vi "GetWL.vi"(2 "error in (no error)":errorcluster, 3 "Integration Time":i32, 4 "Type":enum16{"Get Background", "Measure", "Raw"}(ring)=enum."Measure", 5 "USB4000 Params In":T1) -> (0 "error out":errorcluster, 1 "USB4000 Params Out":T1)   [LabVIEW 2012]
uses:
  Controls/USB4000_Data.ctl
panel:
  out "Array length":i32
  out "EL spectrum":dbl[](array[numeric])
  out "Wavelength":dbl[](array[numeric]) format="%.2f"
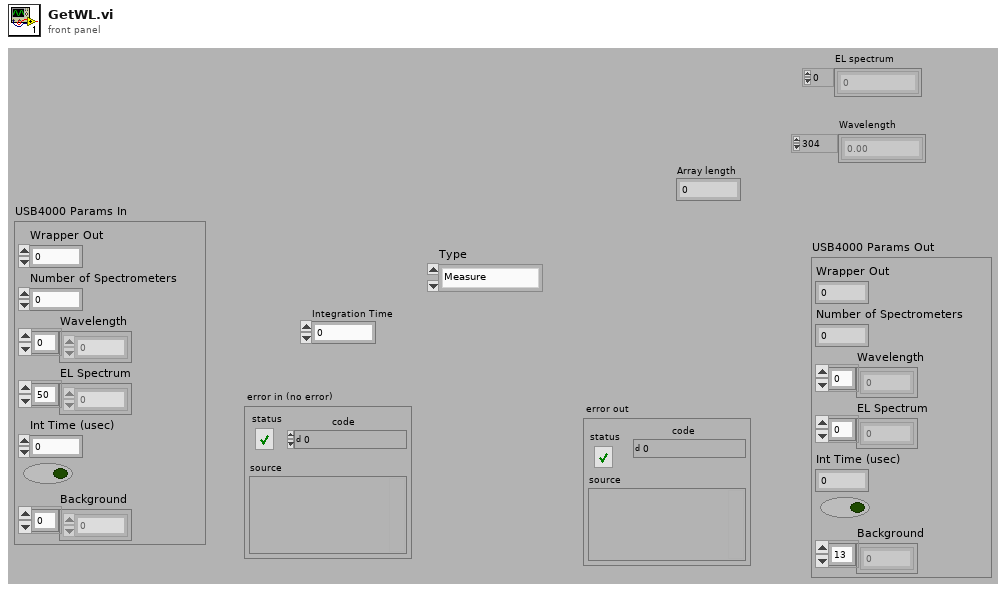
[diagram p1: front panel]
types:
  T1 = typedef "USB4000_Data.ctl" = cluster{"Wrapper Out":u32, "Number of Spectrometers":i32, "Wavelength":dbl[], "EL Spectrum":dbl[], "Int Time (usec)":i32, bool, "Background":dbl[]}
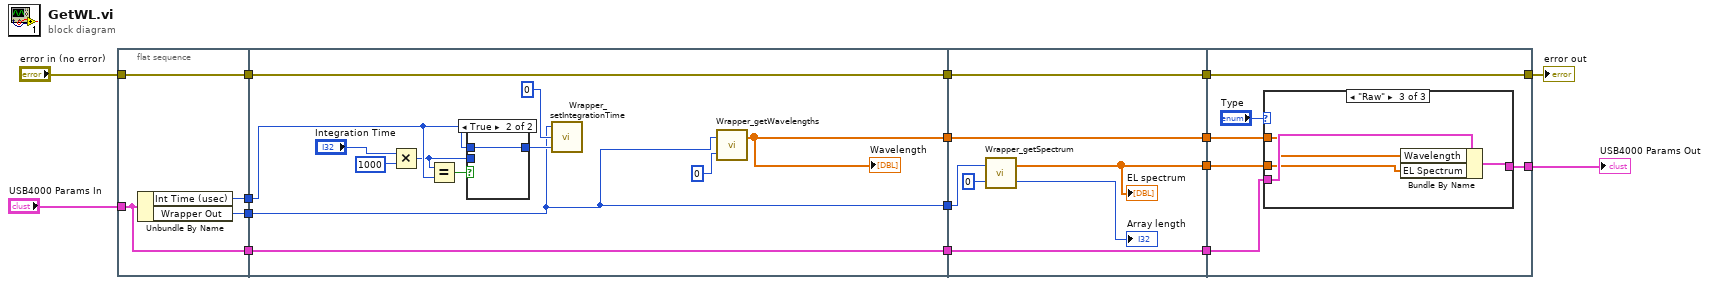
[diagram p0: block diagram]
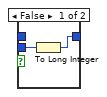
[diagram p2: hidden frame]
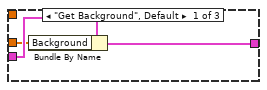
[diagram p3: hidden frame]
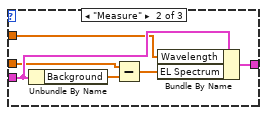
[diagram p4: hidden frame]
diagram:
  n1 = flat-sequence {
    tunnel: "error in (no error)" -> [w17]
    tunnel: [w19] -> w9
    tunnel: [w20] -> w8
    tunnel: [w17] -> w7
    tunnel: "USB4000 Params In" -> [w18]
    tunnel: [w18] -> w3
    tunnel: [w30] -> w16
    tunnel: [w29] -> w12
    tunnel: w9 -> [w21]
    tunnel: w8 -> [w24]
    tunnel: w7 -> [w29]
    tunnel: [w22] -> w4
    tunnel: w3 -> [w22]
    tunnel: [w21] -> w1
    tunnel: w16 -> [w41]
    tunnel: [w41] -> w15
    tunnel: [w37] -> w14
    tunnel: [w40] -> w13
    tunnel: w12 -> [w40]
    tunnel: [w39] -> w5
    tunnel: w4 -> [w39]
    tunnel: w1 -> [w36]
    tunnel: w15 -> [w48]
    tunnel: w14 -> [w47]
    tunnel: w13 -> [w46]
    tunnel: w5 -> [w43]
    tunnel: [w46] -> w2
    tunnel: [w44] -> w10
    frame #0 {
      n2 = Unbundle By Name(w18) -> ("Int Time (usec)"=w20:i32, "Wrapper Out"=w19:u32)
    }
    frame #1 {
      n3 = Multiply(x="Integration Time", y=1000) -> (x*y=w23:i32)
      n4 = Equal?(x=w23, y=w24) -> (x = y?=w26:bool)
      n5 = case shown="True" w26 {
        tunnel: [w33 w35] -> w25
        tunnel: w24 -> [_ w35]
        tunnel: w23 -> [w34 _]
        frame False {
          n6 = To Long Integer(number=w34) -> (32bit integer=w33:i32)
        }
        frame True {
        }
      }
      n7 = call "Wrapper_setIntegrationTime.vi"("Integration Time"=w25, "Index"=0, "Wrapper In"=w21) -> ()  [unwired: 1 out]
      n8 = call "Wrapper_getWavelengths.vi"("Index"=0, "Wrapper"=w21) -> ("WL Values"=w30:dbl[])  [unwired: 1 out]
      "Wavelength" <- w30
    }
    frame #2 {
      n9 = call "Wrapper_getSpectrum.vi"("Index"=0, "Wrapper"=w36) -> ("Length"=→"Array length":i32, "Spectrum Values"=w37:dbl[])
      "EL spectrum" <- w37
    }
    frame #3 {
      n10 = case shown="\"Raw\"" "Type" {
        tunnel: w43 -> [w51 w57 w60]
        tunnel: w48 -> [_ w52 w59]
        tunnel: w47 -> [w50 w55 w58]
        tunnel: [w49 w53 w61] -> w44
        frame "Get Background", Default {
          n11 = Bundle By Name(cluster=w51, "Background"=w50) -> (w49:T1)
        }
        frame "Measure" {
          n12 = Unbundle By Name(w57) -> ("Background"=w56:dbl[])
          n13 = Subtract(x=w55, y=w56) -> (x-y=w54:dbl[])
          n14 = Bundle By Name(cluster=w57, "Wavelength"=w52, "EL Spectrum"=w54) -> (w53:T1)
        }
        frame "Raw" {
          n15 = Bundle By Name(cluster=w60, "Wavelength"=w59, "EL Spectrum"=w58) -> (w61:T1)
        }
      }
    }
  }
  "USB4000 Params Out" <- w10
  "error out" <- w2
